vi "2 MissionHeadingGoodness.vi"(6 "Waypoint in":refnum<class "Waypoint.lvclass">, 7 "Downwind?":bool, 8 "Waypoint Location":T3 {"North" format="%#_10f"; "East" format="%#_8f"}, 9 "Heading\nto Test":T2 format="%05.1f", 10 "UW Tack":dbl, 11 "Into irons?":bool) -> (0 "Pure Waypoint Goodness":dbl, 1 "Direction Change Goodness":dbl, 2 "No-Sail Goodness":dbl, 3 "Target Goodness":dbl, 4 "Pure Wind Goodness":dbl)   [LabVIEW 2011]
doc: "This VI simply takes in a heading to test, runs the necessary component goodness functions and outputs their \"goodness value\" for that heading."
uses:
  2 Typedefs/UTM Location.ctl
  2 Classes/Waypoint/Waypoint.lvclass
  2 Typedefs/heading.ctl
  2 Typedefs/apparent wind direction.ctl
  2 Globals/2 Global.vi
  2 Globals/2 TuningConstants.vi
panel:
  out "Heading Goodness":T1
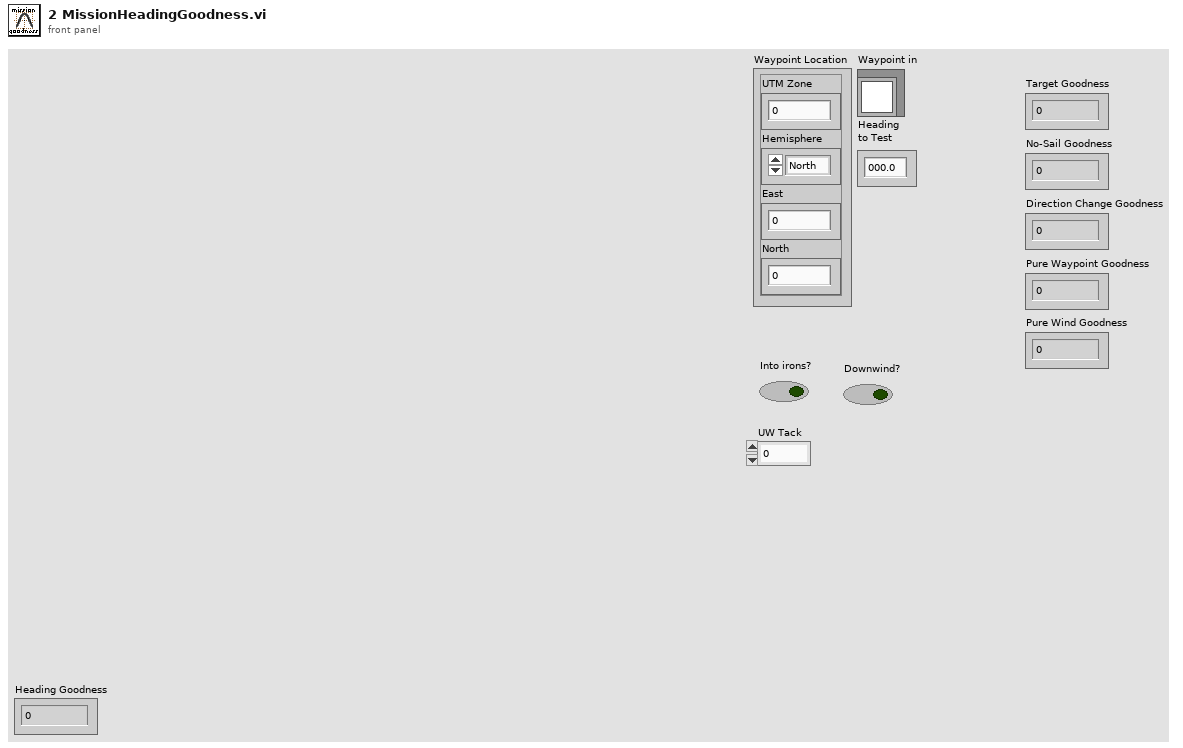
[diagram p1: front panel]
types:
  T1 = typedef "apparent wind direction.ctl" = dbl
  T2 = typedef "heading.ctl" = dbl
  T3 = typedef "UTM Location.ctl" = cluster{"UTM Zone":dbl, "Hemisphere":enum16{"North", "South"}, "East":dbl, "North":dbl}
  T4 = typedef "absolute wind direction.ctl" = dbl
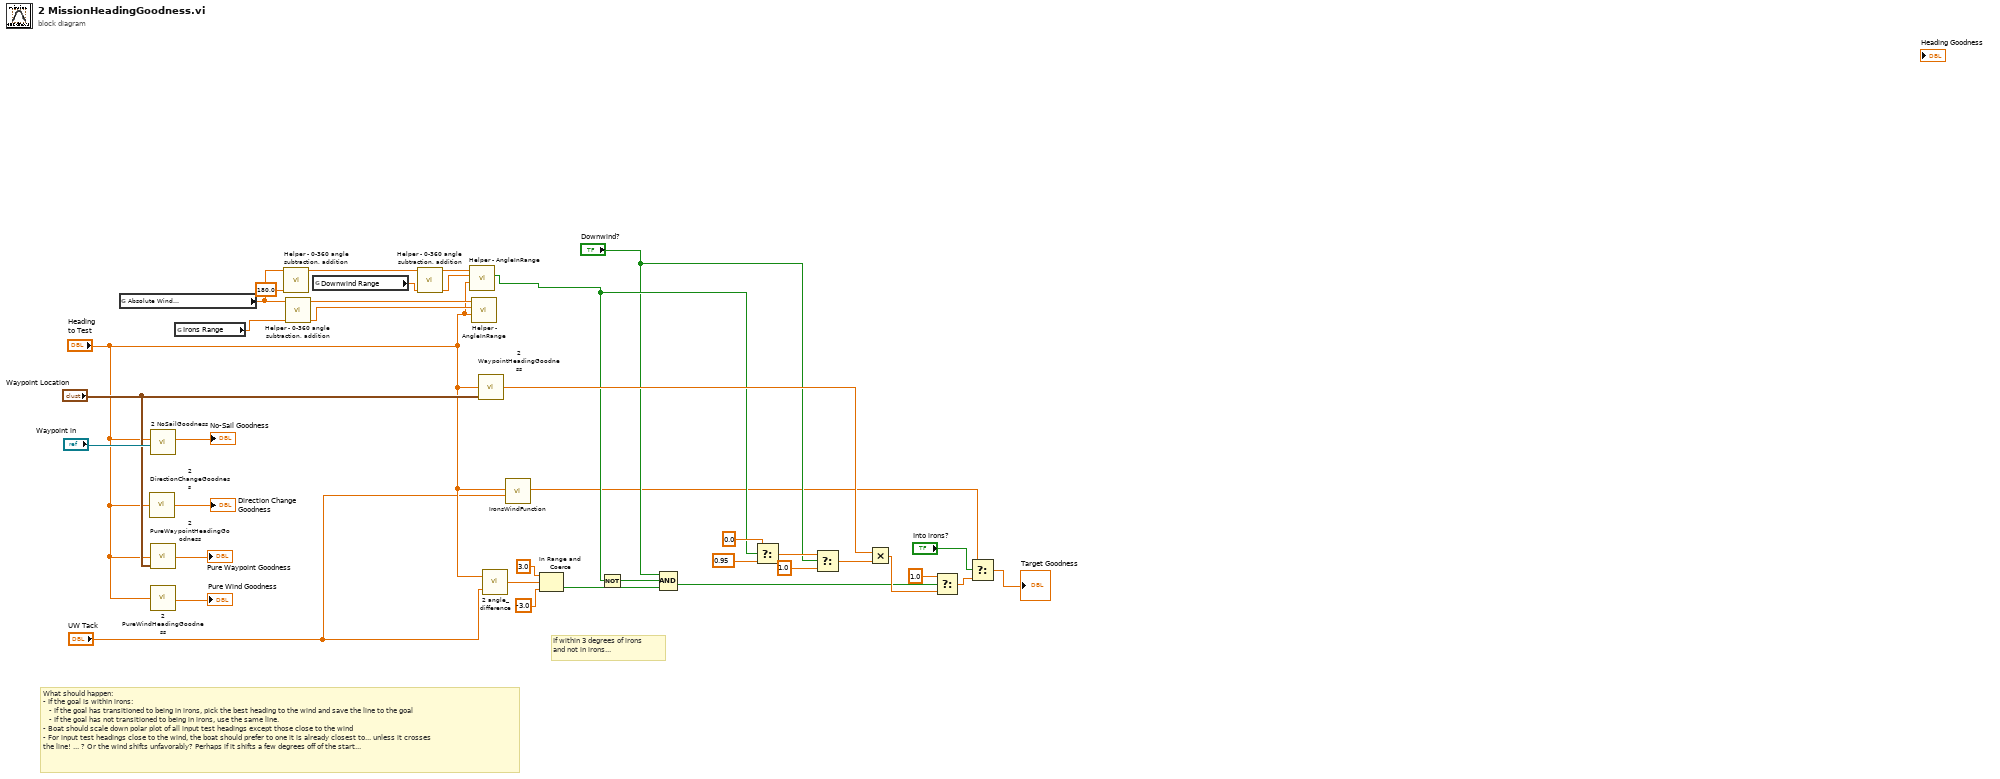
[diagram p0: block diagram]
diagram:
  # "If within 3 degrees of irons\nand not in irons..."
  # "What should happen:\n- If the goal is within irons:\n   - If the goal has transitioned to being in irons, pick the best heading to the wind and save the line to the goal\n   - If the goal has not transitioned to being in irons, use the same line.\n- Boat should scale down polar plot of all input test headings except those close to the wind\n- For input test headings close to the wind, the boat should prefer to one it is already closest to... unless it crosses\nthe line! ... ? Or the wind shifts unfavorably? Perhaps if it shifts a few degrees off of the start..."
  n1 = global read "2 Global.vi" "Absolute Wind\nDirection (º)"() -> (w12:T4)
  n2 = call "2 DirectionChangeGoodness.vi"("Test Heading"="Heading\nto Test") -> ("Goodness"=→"Direction Change Goodness":dbl)
  n3 = call "2 NoSailGoodness.vi"("Waypoint in"="Waypoint in", "Heading to Test"="Heading\nto Test") -> ("Goodness"=→"No-Sail Goodness":dbl)  [unwired: 9 in]
  n4 = call "2 PureWaypointHeadingGoodness.vi"("Waypoint Location"="Waypoint Location", "Heading to Test"="Heading\nto Test") -> ("Goodness"=→"Pure Waypoint Goodness":dbl)  [unwired: 3 in]
  n5 = call "2 PureWindHeadingGoodness.vi"("Heading\nto Test"="Heading\nto Test") -> ("Goodness"=→"Pure Wind Goodness":dbl)  [unwired: 4 in]
  n6 = global read "2 TuningConstants.vi" "Irons Range"() -> (w26:dbl)
  n7 = call "Helper - 0-360 angle subtraction, addition.vi"("y"=180.0, "x"=w12) -> ("x - y"=w10:T1)  [unwired: 8 in, 1 out]
  n8 = call "Helper - 0-360 angle subtraction, addition.vi"("y"=w26, "x"=w12) -> ("x + y"=w24:dbl, "x - y"=w25:T1)  [unwired: 8 in]
  n9 = global read "2 TuningConstants.vi" "Downwind Range"() -> (w9:dbl)
  n10 = call "Helper - 0-360 angle subtraction, addition.vi"("y"=w9, "x"=w10) -> ("x + y"=w14:dbl, "x - y"=w13:T1)  [unwired: 8 in]
  n11 = call "Helper - AngleInRange.vi"("Angle to check"="Heading\nto Test", "Angle 2"=w14, "Angle 1"=w13) -> ("In range?"=w8:bool)  [unwired: 8 in]
  n12 = call "Helper - AngleInRange.vi"("Angle to check"="Heading\nto Test", "Angle 2"=w24, "Angle 1"=w25) -> ()  [unwired: 8 in, 1 out]
  n13 = call "2 WaypointHeadingGoodness.vi"("Waypoint Location"="Waypoint Location", "Heading\nto Test"="Heading\nto Test") -> ("Goodness"=w21:dbl)  [unwired: 3 in]
  n14 = call "2 angle_difference.vi"("Angle 2"="UW Tack", "Angle 1"="Heading\nto Test") -> ("Difference"=w30:dbl)
  n15 = call "IronsWindFunction.vi"("Desired Irons Angle"="UW Tack", "Angle to test"="Heading\nto Test") -> ("Goodness"=w3:dbl)  [unwired: 9 in]
  n16 = In Range and Coerce(upper limit=T1 3.0, x=w30, lower limit=T1 -3.0) -> (In Range?=w17:bool)  [unwired: 1 out]
  n17 = Not(x=w8) -> (.not. x?=w16:bool)
  n18 = Compound Arithmetic op=AND("Downwind?", w16, w17) -> (w15:bool)
  n19 = Select(t=0.0, s=w8, f=0.95 ("t")) -> (s? t:f=w23:dbl)
  n20 = Select(t=w23, s="Downwind?", f=1.0 ("t")) -> (s? t:f=w27:dbl)
  n21 = Multiply(x=w21, y=w27) -> (x*y=w19:dbl)
  n22 = Select(t=1.0, s=w15, f=w19) -> (s? t:f=w5:dbl)
  n23 = Select(t=w3, s="Into irons?", f=w5) -> (s? t:f=→"Target Goodness":dbl)
